vi "remove class extension.vi"(11 "class name in":string) -> (3 "class name out":string)   [LabVIEW 2018, in "LV-ORM.lvclass"]
uses:
  LV-ORM.lvclass
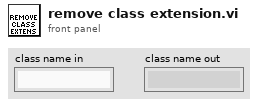
[diagram p1: front panel]
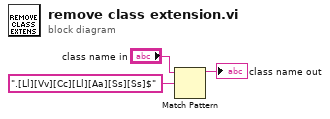
[diagram p0: block diagram]
diagram:
  n1 = Match Pattern(string="class name in", regular expression=".[Ll][Vv][Cc][Ll][Aa][Ss][Ss]$") -> (before substring=→"class name out":string)  [unwired: 1 in, 3 out]
